vi "dfd_Group Delay_Gradient.vi"(10 "Coefficients":cluster{"r":dbl[], "theta":dbl[], "offset":dbl}, 11 "Design Info":T1={"p"=2, "freq grid"=[], "d"=[], "weight"=[], "Order"=0, "radius"=0.0}) -> (1 "Error":dbl, 2 "Coefficients (dup)":cluster{"r":dbl[], "theta":dbl[], "offset":dbl}, 3 "Design Info (dup)":T1={"p"=2, "freq grid"=[], "d"=[], "weight"=[], "Order"=0, "radius"=0.0}, 4 "Gradients":cluster{"r":dbl[], "theta":dbl[], "offset":dbl})   [LabVIEW 2017, in "NI_DigFilter_Design.lvlib"]
uses:
  <vilib>/addons/Digital Filter Design/NI_DigFilter_Design.lvlib
  <vilib>/addons/Digital Filter Design/_GroupDelay.llb/dfd_Group Delay_Design Info.ctl
  <vilib>/Analysis/baseanly.llb/Real A x B.vi
  <vilib>/Analysis/NI_AALBase.lvlib
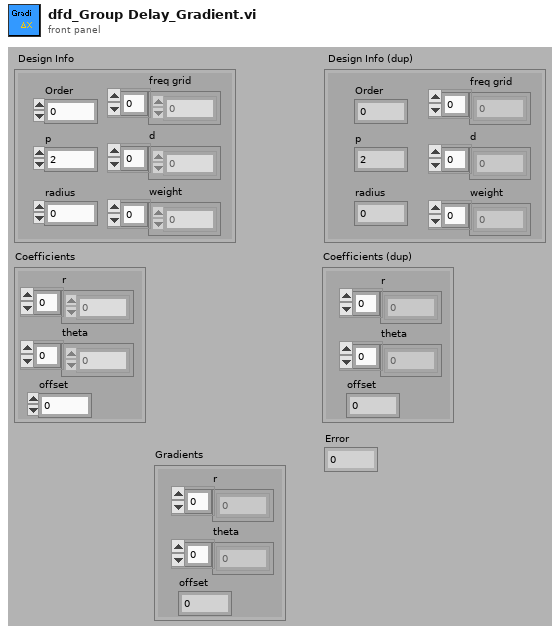
[diagram p1: front panel]
types:
  T1 = typedef "dfd_Group Delay_Design Info.ctl" = cluster{"p":i32, "freq grid":dbl[], "d":dbl[], "weight":dbl[], "Order":i32, "radius":dbl}
  T2 = typedef "NI_Matrix.lvlib/RealMatrix.ctl" = dbl[][]
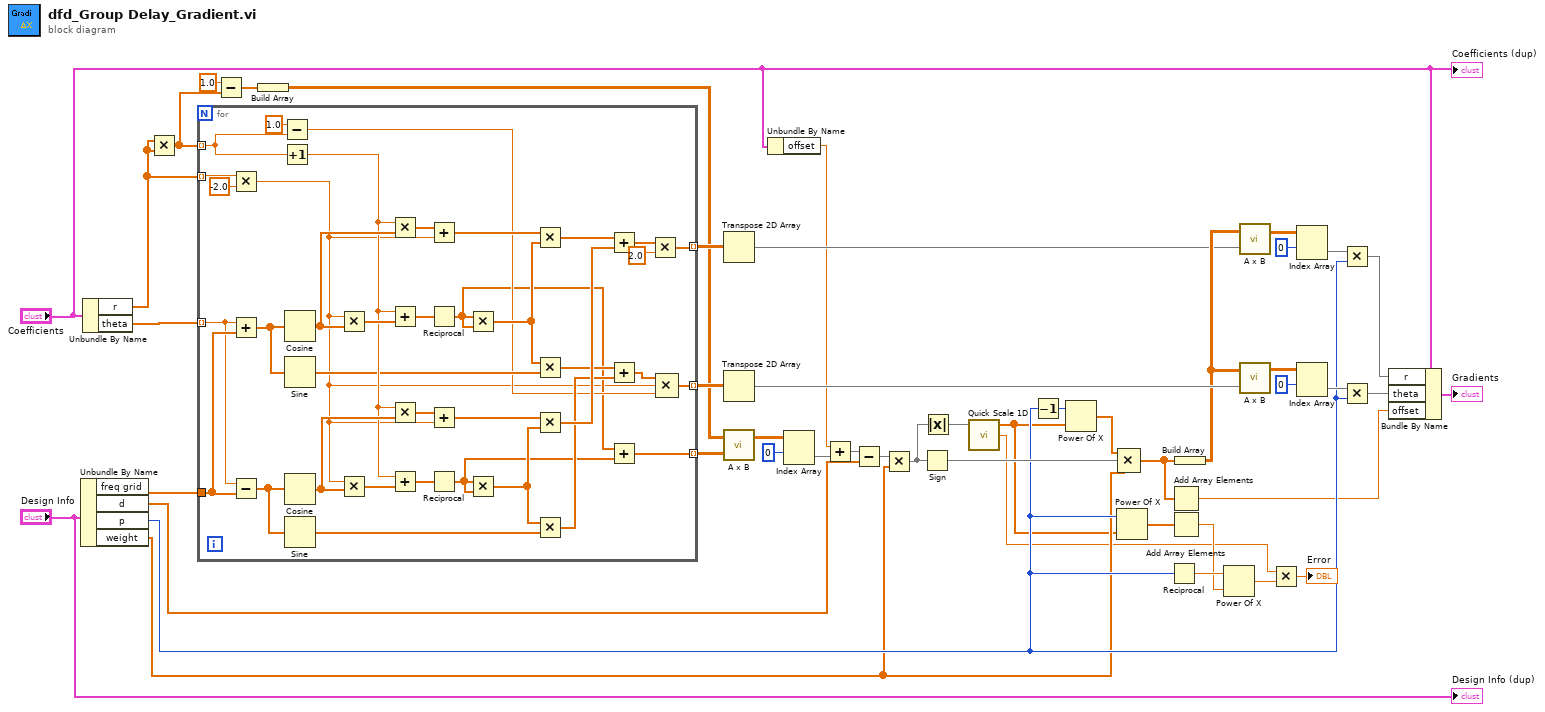
[diagram p0: block diagram]
diagram:
  n1 = Unbundle By Name("Design Info") -> ("freq grid"=w23:dbl[], "d"=w20:dbl[], "p"=w27:i32, "weight"=w15:dbl[])
  n2 = Unbundle By Name("Coefficients") -> ("r"=w10:dbl[], "theta"=w29:dbl[])
  n3 = Multiply(x=w10, y=w10) -> (x*y=w6:dbl[])
  n4 = for {
    tunnel: w29 -> [w83] mode=indexing
    tunnel: w23 -> [w84]
    tunnel: [w54] -> w40 mode=indexing
    tunnel: [w66] -> w44 mode=indexing
    tunnel: [w55] -> w39 mode=indexing
    tunnel: w10 -> [w52] mode=indexing
    tunnel: w6 -> [w51] mode=indexing
    n5 = Multiply(x=w52, y=-2.0) -> (x*y=w48:dbl)
    n6 = Add(x=w83, y=w84) -> (x+y=w73:dbl[])
    n7 = Subtract(x=w83, y=w84) -> (x-y=w72:dbl[])
    n8 = Subtract(x=1.0, y=w51) -> (x-y=w57:dbl)
    n9 = Increment(x=w51) -> (x+1=w71:dbl)
    n10 = Cosine(x=w73) -> (cos(x)=w76:dbl[])
    n11 = Sine(x=w73) -> (sin(x)=w63:dbl[])
    n12 = Cosine(x=w72) -> (cos(x)=w77:dbl[])
    n13 = Sine(x=w72) -> (sin(x)=w61:dbl[])
    n14 = Multiply(x=w48, y=w76) -> (x*y=w80:dbl[])
    n15 = Multiply(x=w48, y=w77) -> (x*y=w81:dbl[])
    n16 = Multiply(x=w71, y=w76) -> (x*y=w75:dbl[])
    n17 = Add(x=w71, y=w80) -> (x+y=w68:dbl[])
    n18 = Multiply(x=w71, y=w77) -> (x*y=w74:dbl[])
    n19 = Add(x=w71, y=w81) -> (x+y=w67:dbl[])
    n20 = Add(x=w75, y=w48) -> (x+y=w65:dbl[])
    n21 = Reciprocal(x=w68) -> (1/x=w49:dbl[])
    n22 = Add(x=w74, y=w48) -> (x+y=w64:dbl[])
    n23 = Reciprocal(x=w67) -> (1/x=w50:dbl[])
    n24 = Multiply(x=w49, y=w49) -> (x*y=w62:dbl[])
    n25 = Multiply(x=w50, y=w50) -> (x*y=w60:dbl[])
    n26 = Multiply(x=w65, y=w62) -> (x*y=w70:dbl[])
    n27 = Multiply(x=w62, y=w63) -> (x*y=w59:dbl[])
    n28 = Multiply(x=w64, y=w60) -> (x*y=w69:dbl[])
    n29 = Multiply(x=w60, y=w61) -> (x*y=w58:dbl[])
    n30 = Add(x=w70, y=w69) -> (x+y=w79:dbl[])
    n31 = Add(x=w59, y=w58) -> (x+y=w56:dbl[])
    n32 = Add(x=w49, y=w50) -> (x+y=w66:dbl[])
    n33 = Multiply(x=w79, y=2.0) -> (x*y=w54:dbl[])
    n34 = Compound Arithmetic op=MULTIPLY(w56, w48, w57) -> (w55:dbl[])
  }
  n35 = Subtract(x=1.0, y=w6) -> (x-y=w8:dbl[])
  n36 = Build Array(w8) -> (w7:dbl[][])
  n37 = Transpose 2D Array(2D array=w40) -> (transposed array=w36:dbl[][])
  n38 = Transpose 2D Array(2D array=w39) -> (transposed array=w38:dbl[][])
  n39 = call-poly <vilib>:"A x B.vi"("B"=w44, "A"=w7) -> ("A x B"=w46:T2)  [unwired: 1 out]
  n40 = Unbundle By Name("Coefficients") -> ("offset"=w18:dbl)
  n41 = Index Array(array=w46, index (row)=0) -> (element=w43:dbl[])  [unwired: 1 in]
  n42 = Add(x=w18, y=w43) -> (x+y=w19:dbl[])
  n43 = Subtract(x=w19, y=w20) -> (x-y=w16:dbl[])
  n44 = Multiply(x=w16, y=w15) -> (x*y=w17:dbl[])
  n45 = Sign(1:w17) -> (0:w41:dbl[])
  n46 = Absolute Value(x=w17) -> (abs(x)=w5:dbl[])
  n47 = call <vilib>:"Quick Scale 1D.vi"("X"=w5) -> ("Y[i]=X[i]/Max|X|"=w4:dbl[], "max|X|"=w3:dbl)  [unwired: 1 out]
  n48 = Decrement(x=w27) -> (x-1=w28:i32)
  n49 = Power Of X(1:w4, 2:w28) -> (0:w42:dbl[])
  n50 = Power Of X(1:w4, 2:w27) -> (0:w14:dbl[])
  n51 = Compound Arithmetic op=MULTIPLY(w42, w41, w15) -> (w22:dbl[])
  n52 = Reciprocal(x=w27) -> (1/x=w26:dbl)
  n53 = Add Array Elements(numeric array=w22) -> (sum=w21:dbl)
  n54 = Add Array Elements(numeric array=w14) -> (sum=w25:dbl)
  n55 = Build Array(w22) -> (w37:dbl[][])
  n56 = Power Of X(1:w25, 2:w26) -> (0:w11:dbl)
  n57 = call-poly <vilib>:"A x B.vi"("B"=w36, "A"=w37) -> ("A x B"=w33:T2)  [unwired: 1 out]
  n58 = call-poly <vilib>:"A x B.vi"("B"=w38, "A"=w37) -> ("A x B"=w31:T2)  [unwired: 1 out]
  n59 = Multiply(x=w3, y=w11) -> (x*y=→"Error":dbl)
  n60 = Index Array(array=w33, index (row)=0) -> (element=w32:dbl[])  [unwired: 1 in]
  n61 = Index Array(array=w31, index (row)=0) -> (element=w30:dbl[])  [unwired: 1 in]
  n62 = Multiply(x=w32, y=w27) -> (x*y=w13:dbl[])
  n63 = Multiply(x=w30, y=w27) -> (x*y=w24:dbl[])
  n64 = Bundle By Name(cluster="Coefficients", "r"=w13, "theta"=w24, "offset"=w21) -> (→"Gradients":cluster{"r":dbl[], "theta":dbl[], "offset":dbl})
  "Design Info (dup)" <- "Design Info"
  "Coefficients (dup)" <- "Coefficients"
